vi "Listfiles Example.vi"(8 "Error In":errorcluster) -> (0 "error out":errorcluster)   [LabVIEW 2014]
doc: "Tested with:\n - Arduino Nano\n - Wemos D1 with ESP8266\n\nOutput of this VI in simulation folder is recursive list of files.\nRunning OK on Wemos D1 because it has enough RAM, on Arduino Nano it can write just few first dirs due to small RAM.\nIf run on desktop PC it can list long list of files, because in root dir there is .git dir"
uses:
  <vilib>/LabVIEW Universal Transcriptor/LabVIEW to Arduino Transcriptor/Transcriptors/System API/Serial println string.vi
  <vilib>/LabVIEW Universal Transcriptor/LabVIEW Universal Transcriptor SD Card Library/LabVIEW Universal Transcriptor SD Card Library.lvlib
  <vilib>/LabVIEW Universal Transcriptor/LabVIEW to Arduino Transcriptor/Transcriptors/System API/System Serial Library Variables/System Serial Library Variables.lvlib
panel:
  out "String Buffer":string
  # "Tested with:\n  - Arduino Nano\n  - Wemos D1 with ESP8266\n\nOutput of this VI in simulation folder is recursive list of files.\nRunning OK on Wemos D1 because it has enough RAM, on Arduino Nano it can write just few first dirs due to small RAM.\nIf run on desktop PC it can list long list of files, because in root dir there is .git dir"
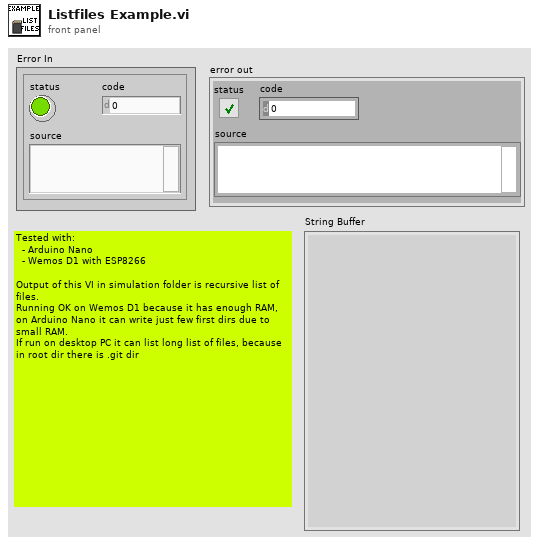
[diagram p1: front panel]
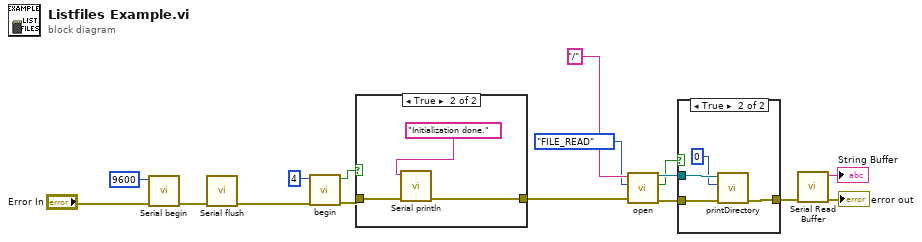
[diagram p0: block diagram]
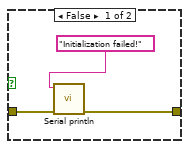
[diagram p3: hidden frame]
diagram:
  n1 = call <vilib>:"Serial begin.vi"("Error In"="Error In", "speed (Bd)"=9600) -> ("Error Out"=w3:errorcluster)  [unwired: 9 in]
  n2 = call <vilib>:"Serial flush.vi"("Error In"=w3) -> ("Error Out"=w2:errorcluster)  [unwired: 10 in]
  n3 = call <vilib>:"begin.vi"("Error In"=w2, "CS pin (optional)"=u8 4) -> ("Error Out"=w13:errorcluster, "success?"=w12:bool)  [unwired: 8 in]
  n4 = case shown="True" w12 {
    tunnel: w13 -> [w18 w21]
    tunnel: [w17 w20] -> w11
    frame False {
      n5 = call-poly <vilib>:"Serial println.vi"("Error In"=w18, "string in"="Initialization failed!" ("filepath")) -> ("Error Out"=w17:errorcluster)  [unwired: 9 in]
    }
    frame True {
      n6 = call-poly <vilib>:"Serial println.vi"("Error In"=w21, "string in"="Initialization done." ("filepath")) -> ("Error Out"=w20:errorcluster)  [unwired: 9 in]
    }
  }
  n7 = call <vilib>:"open.vi"("Error In"=w11, "mode"=enum16{"FILE_READ", "FILE_WRITE"}."FILE_READ", "filepath"="/") -> ("Error Out"=w8:errorcluster, "opened?"=w1:bool, "File out"=w7:refnum<class "File.lvclass">)  [unwired: 6 in]
  n8 = case shown="True" w1 {
    tunnel: w8 -> [w23 w27]
    tunnel: w7 -> [_ w26]
    tunnel: [w23 w24] -> w6
    frame False {
    }
    frame True {
      n9 = call <vilib>:"printDirectory.vi"("Error In"=w27, "nested level"=u8 0, "file"=w26) -> ("Error Out"=w24:errorcluster)  [unwired: 8 in]
    }
  }
  n10 = call <vilib>:"Serial Read Buffer.vi"("Error In"=w6) -> ("Error Out"=→"error out":errorcluster, "String Buffer"=→"String Buffer":string)  [unwired: 9 in]
